vi "read out current z.vi"() -> ()   [LabVIEW 2018]
panel:
  in  "read count":i32=100
  out "current z (steps)":string="where z"
  in  "ASI stage VISA resource name":refnum<visa-resource-name>="COM5"
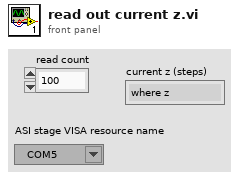
[diagram p1: front panel]
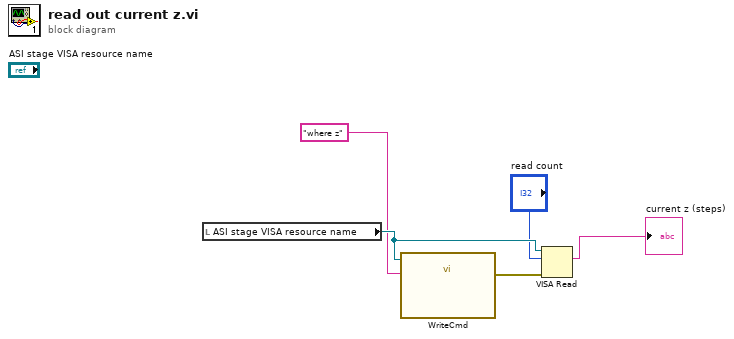
[diagram p0: block diagram]
diagram:
  n1 = local read "ASI stage VISA resource name"() -> (w5:refnum<visa-resource-name>)
  n2 = call "WriteCmd.vi"("Command"="where z", "VISA resource name"=w5) -> ("error"=w4:errorcluster)  [unwired: 1 in]
  n3 = VISA Read(VISA resource name=w5, byte count="read count", error in (no error)=w4) -> (read buffer=→"current z (steps)":string)  [unwired: 3 out]
